vi "VISA resource.vi"() -> ()   [LabVIEW 2021]
panel:
  in  "VISA resource":refnum<visa-resource-name>
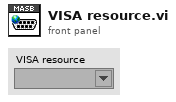
[diagram p1: front panel]
diagram:
